vi "StateToLegVelocity.vi"(9 "ControlParams":T1, 10 "State":dbl[](array[numeric])) -> (2 "Vr":i16, 3 "Vl":i16)   [LabVIEW 2011]
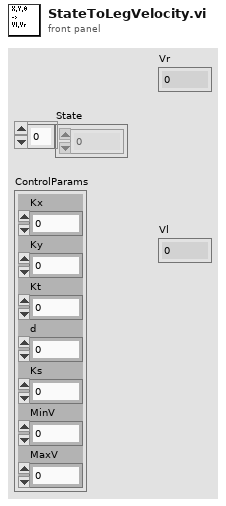
[diagram p1: front panel]
types:
  T1 = cluster{"Kx":dbl, "Ky":dbl, "Kt":dbl, "d":dbl, "Ks":dbl, "MinV":i16, "MaxV":i16}
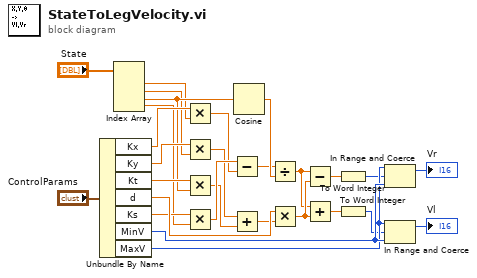
[diagram p0: block diagram]
diagram:
  n1 = Unbundle By Name("ControlParams") -> ("Kx"=w20:dbl, "Ky"=w21:dbl, "Kt"=w22:dbl, "d"=w24:dbl, "Ks"=w23:dbl, "MinV"=w28:i16, "MaxV"=w27:i16)
  n2 = Index Array(array="State") -> (element #1=w15:dbl, element #2=w16:dbl, element #3=w17:dbl, element #4=w1:dbl)  [unwired: 4 in]
  n3 = Multiply(x=w20, y=w15) -> (x*y=w2:dbl)
  n4 = Multiply(x=w21, y=w16) -> (x*y=w5:dbl)
  n5 = Multiply(x=w22, y=w17) -> (x*y=w6:dbl)
  n6 = Multiply(x=w23, y=w1) -> (x*y=w10:dbl)
  n7 = Subtract(x=w10, y=w2) -> (x-y=w3:dbl)
  n8 = Add(x=w5, y=w6) -> (x+y=w8:dbl)
  n9 = Cosine(x=w17) -> (cos(x)=w4:dbl)
  n10 = Divide(x=w3, y=w4) -> (x/y=w7:dbl)
  n11 = Multiply(x=w24, y=w8) -> (x*y=w9:dbl)
  n12 = Subtract(x=w7, y=w9) -> (x-y=w26:dbl)
  n13 = Add(x=w7, y=w9) -> (x+y=w25:dbl)
  n14 = To Word Integer(number=w26) -> (16bit integer=w11:i16)
  n15 = To Word Integer(number=w25) -> (16bit integer=w12:i16)
  n16 = In Range and Coerce(upper limit=w27, x=w11, lower limit=w28) -> (coerced(x)=→"Vr":i16)  [unwired: 1 out]
  n17 = In Range and Coerce(upper limit=w27, x=w12, lower limit=w28) -> (coerced(x)=→"Vl":i16)  [unwired: 1 out]
